vi "Load Specs Timing Levels to Sessions.vi"(0 "sequence context":refnum<k7>, 5 "specification file paths":string[](array[string]), 7 "levels file paths":string[](array[string]), 9 "timing file paths":string[](array[string]), 11 "error in":errorcluster) -> (15 "error out":errorcluster)   [LabVIEW 2020, in "NIDigitalSPI.lvlib"]
uses:
  NIDigitalSPI.lvlib
  <instrlib>/niDigital/niDigital.llb/niDigital Load Specifications Levels and Timing (Multiple).vi
  <vilib>/Plug-In SDKs/Clients/Session Management V1/Session Reservation/Session Reservation.lvclass
  <vilib>/Plug-In SDKs/Sessions/niDigital/NI Session Management niDigital.lvlib
  <vilib>/Plug-In SDKs/Clients/Session Management V1/Session Reservation/Initialize and Close Session Behavior.ctl
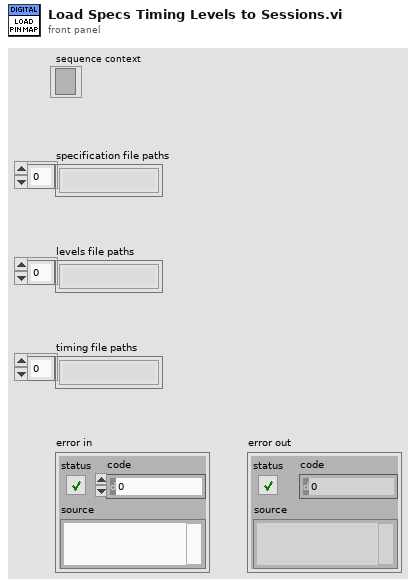
[diagram p1: front panel]
types:
  T1 = typedef "NI Session Management V1 Client.lvlib/Session Reservation.lvclass/Initialize and Close Session Behavior.ctl" = enum16{"Auto", "Initialize and Close", "Attach and Detach", "Initialize and Detach", "Attach and Close"}
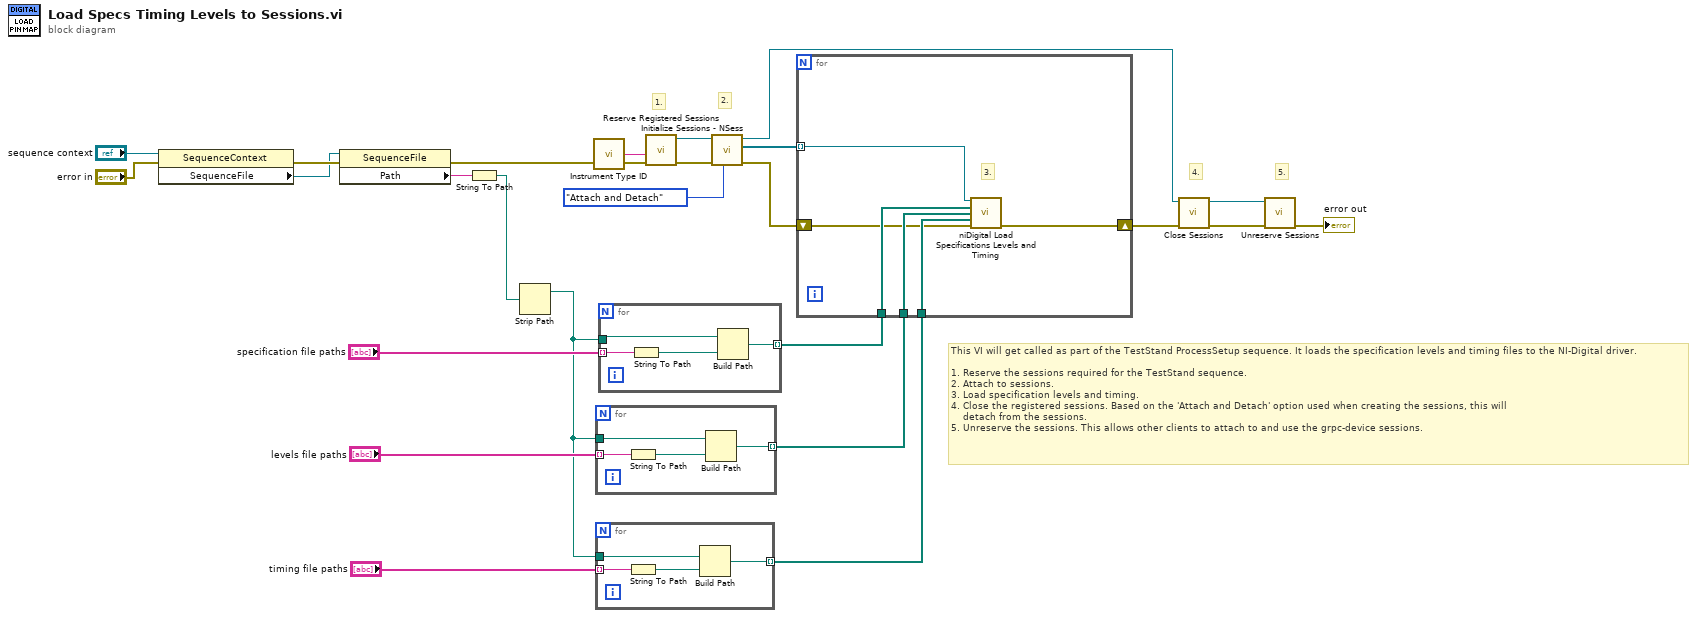
[diagram p0: block diagram]
diagram:
  # "5."
  # "4."
  # "2."
  # "1."
  # "This VI will get called as part of the TestStand ProcessSetup sequence. It loads the specification levels and timing files to the NI-Digital driver.\n\n1. Reserve the sessions required for the TestStand sequence.\n2. Attach to sessions.\n3. Load specification levels and timing.\n4. Close the registered sessions. Based on the 'Attach and Detach' option used when creating the sessions, this will\n    detach from the sessions.\n5. Unreserve the sessions. This allows other clients to attach to and use the grpc-device sessions."
  n1 = property class="SequenceContext"(reference="sequence context", error in="error in") -> (error out=w18:errorcluster, "SequenceFile"=w16:refnum<k7>)  [unwired: 1 out]
  n2 = property class="SequenceFile"(reference=w16, error in=w18) -> (error out=w8:errorcluster, "Path"=w15:string)  [unwired: 1 out]
  n3 = String To Path(string=w15) -> (path=w14:path)
  n4 = Strip Path(path=w14) -> (stripped path=w13:path)  [unwired: 1 out]
  n5 = call <vilib>:"Instrument Type ID.vi"() -> ("instrument type id"=w6:string)  [unwired: 5 in]
  n6 = for {
    tunnel: "levels file paths" -> [w29] mode=indexing
    tunnel: [w28] -> w21 mode=indexing
    tunnel: w13 -> [w26]
    n7 = String To Path(string=w29) -> (path=w27:path)
    n8 = Build Path(base path=w26, name or relative path=w27) -> (appended path=w28:path)
  }
  n9 = for {
    tunnel: "timing file paths" -> [w33] mode=indexing
    tunnel: [w31] -> w20 mode=indexing
    tunnel: w13 -> [w30]
    n10 = String To Path(string=w33) -> (path=w32:path)
    n11 = Build Path(base path=w30, name or relative path=w32) -> (appended path=w31:path)
  }
  n12 = for {
    tunnel: "specification file paths" -> [w37] mode=indexing
    tunnel: [w34] -> w22 mode=indexing
    tunnel: w13 -> [w36]
    n13 = String To Path(string=w37) -> (path=w35:path)
    n14 = Build Path(base path=w36, name or relative path=w35) -> (appended path=w34:path)
  }
  n15 = call <vilib>:"Reserve Registered Sessions.vi"("error in"=w8, "instrument type id"=w6) -> ("error out"=w12:errorcluster, "session reservation out"=w11:refnum<class "Session Reservation.lvclass">)  [unwired: 8 in]
  n16 = call <vilib>:"Initialize Sessions - NSess.vi"("initialize and close session behavior"=Initialize_and_Close_Session_Behavior."Attach and Detach", "error in"=w12, "session reservation in"=w11) -> ("error out"=w9:errorcluster, "sessions"=w10:refnum<k15>[], "session reservation out"=w1:refnum<class "Session Reservation.lvclass">)  [unwired: 5 in, 1 out]
  n17 = for {
    shift-right: [w38] -> w4
    shift-left: w9 -> [w40]
    tunnel: w22 -> [w43]
    tunnel: w21 -> [w42]
    tunnel: w20 -> [w41]
    tunnel: w10 -> [w39] mode=indexing
    # "3."
    n18 = call-poly <instrlib>:"niDigital Load Specifications Levels and Timing.vi"("instrument handle"=w39, "specifications file paths"=w43, "levels file paths"=w42, "timing file paths"=w41, "error in"=w40) -> ("error out"=w38:errorcluster)  [unwired: 9 in, 1 out]
  }
  n19 = call <vilib>:"Close Sessions.vi"("error in"=w4, "session reservation in"=w1) -> ("error out"=w3:errorcluster, "session reservation out"=w2:refnum<class "Session Reservation.lvclass">)  [unwired: 8 in]
  n20 = call <vilib>:"Unreserve Sessions.vi"("error in"=w3, "session reservation in"=w2) -> ("error out"=→"error out":errorcluster)  [unwired: 9 in]
